vi "BASE_I_O_Screen.vi"(8 "error in (no error)":errorcluster) -> (0 "error out":errorcluster)   [LabVIEW 2017]
doc: "This vi is for manually turn ON and OFF also monitor Output of PLCS. So this is manual screen."
uses:
  <vilib>/Utility/file.llb/Read Delimited Spreadsheet (string).vi
  Global/PLC_to_Auto.vi
panel:
  out "CARD 8 OUTPUT":T1
  out "X27-SPARE 2":bool
  out "X26-SPARE 2":bool
  out "Y22 2":bool
  out "Y25":bool
  out "Y23":bool
  out "Y22":bool
  out "Y21":bool
  out "Y20-SPARE":bool
  out "X27-SPARE":bool
  out "X26-SPARE":bool
  out "X25-REJECTION FULL SENSOR":bool
  out "X24-REJECTION SENSOR":bool
  out "X23-DOOR 4":bool
  out "X22-DOOR 3":bool
  out "PART CLAMP END RS":bool
  out "UP DOWN CYL END RS":bool
  out "UP DOWN CYL  HM RS":bool
  out "PUSHER END RS":bool
  out "PUSHER HM RS":bool
  out "THREAD LOCKER CYL COMPLETE":bool
  out "SHUTTLE OPEN CHECK SENSOR-X300":bool
  out "SPARE":bool
  out "DOOR 2":bool
  out "DOOR 1":bool
  out "SAFETY SENSOR":bool
  out "GREEN LAMP":bool
  out "PRESSURE SWITCH":bool
  out "RESET PB":bool
  out "EMG STOP":bool
  out "CYCLE START TOUCH BUTTON 2":bool
  out "CYCLE START TOUCH BUTTON 1":bool
  out "BUZZER":bool
  out "RED LAMP":bool
  out "UP DN CYL REV SOL":bool
  out "UP DN CYL FWD SOL":bool
  out "PUSHER REV SOL":bool
  out "PUSHER FWD SOL":bool
  out "THREAD LOCKER OFF":bool
  out "THREAD LOCKER ON":bool
  out "PART CLAMP SOL":bool
  in  "Back":bool
  # "I/O Screen"
  # "OUTPUT"
  # "INPUT"
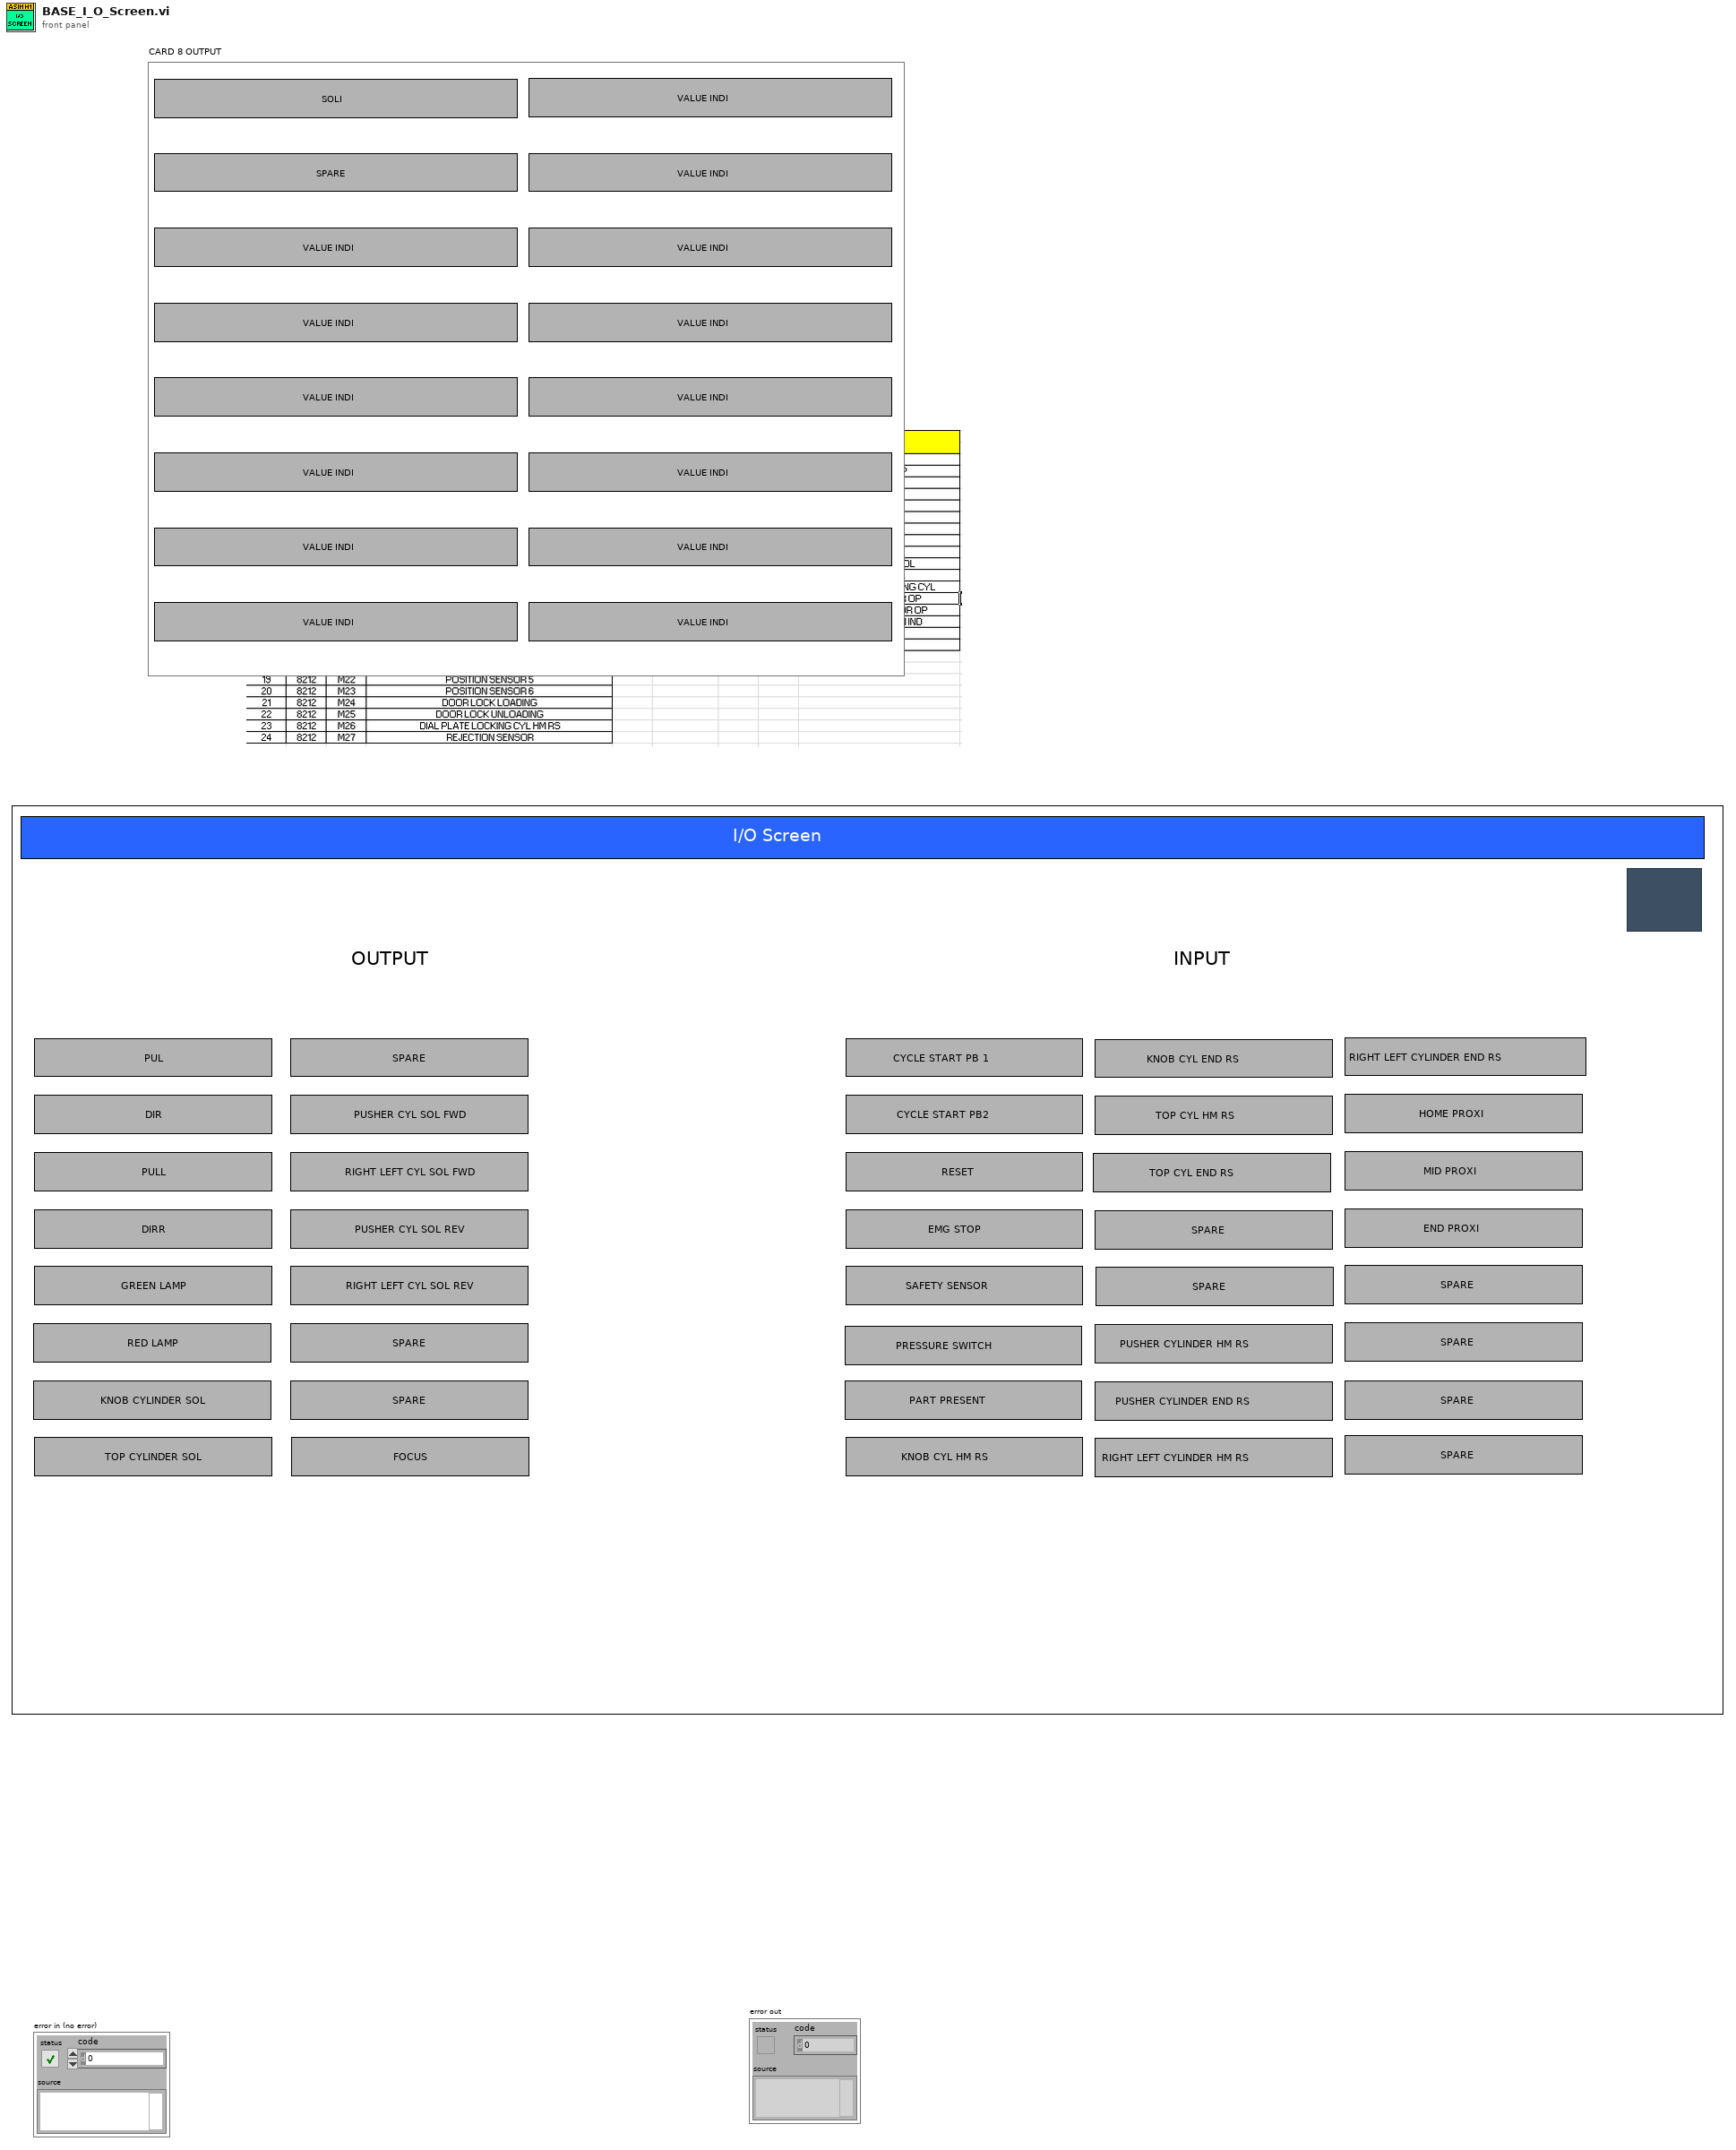
[diagram p1: front panel]
types:
  T1 = cluster{"8 CARD 1":bool, "8 CARD 2":bool, "8 CARD 3":bool, "8 CARD 4":bool, "8 CARD 5":bool, "8 CARD 6":bool, "8 CARD 7":bool, "8 CARD 8":bool, "8 CARD 9":bool, "8 CARD 10":bool, "8 CARD 11":bool, "8 CARD 12":bool, "8 CARD 13":bool, "8 CARD 14":bool, "8 CARD 15":bool, "8 CARD 16":bool}
  T2 = enum32{"invalid app kind", "Development System", "Run Time System", "Student Edition", "Embedded LabVIEW", "Evaluation", "Custom"}
  T3 = enum32{"Invalid", "Standard", "Closed", "Hidden", "Minimized", "Maximized"}
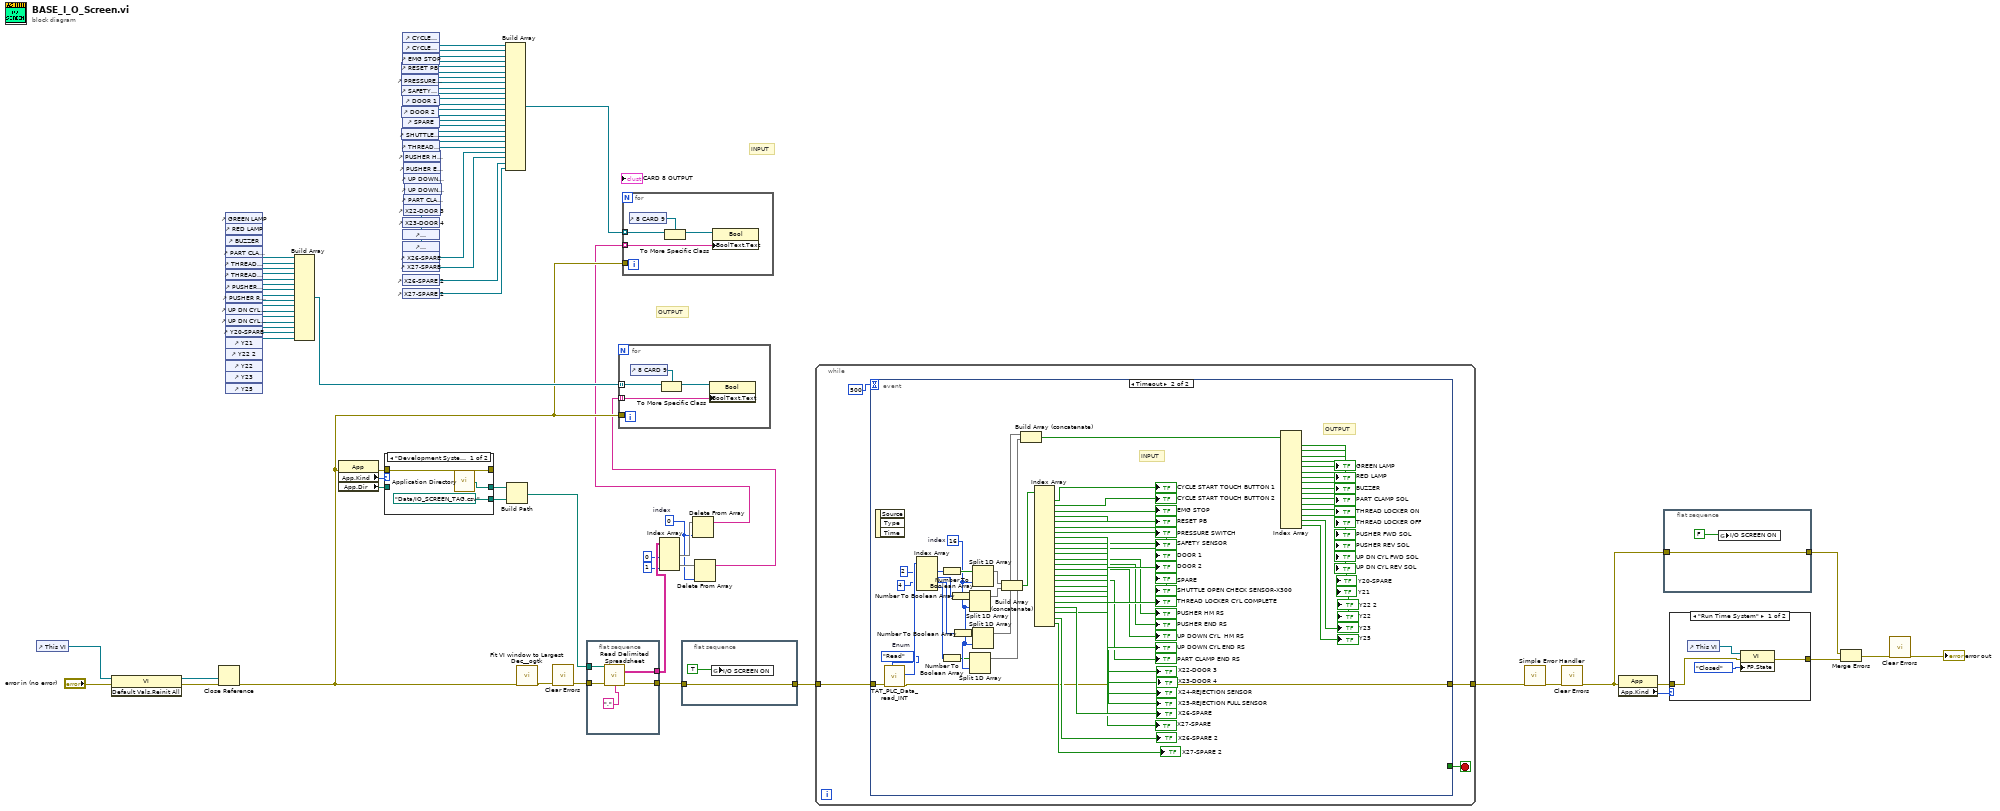
[diagram p0: block diagram]
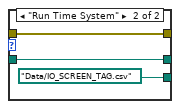
[diagram p2: hidden frame]
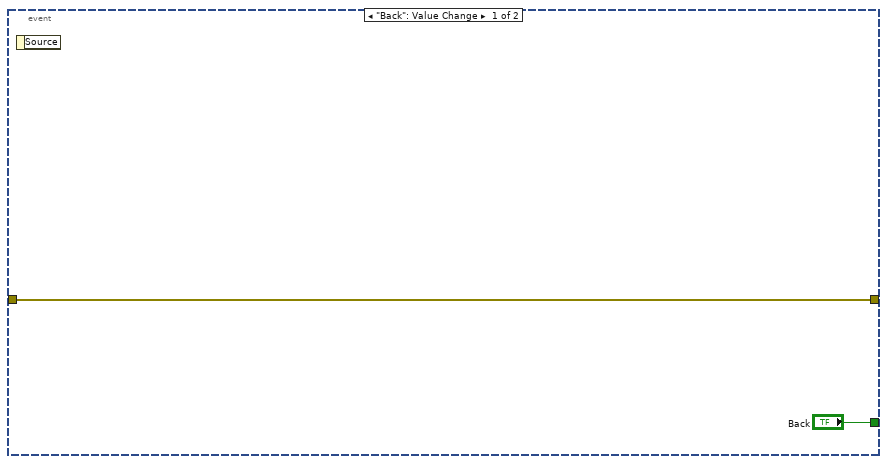
[diagram p4: hidden frame]
diagram:
  w55 = 0  # index
  # "OUTPUT"
  # "INPUT"
  n1 = control-ref of="This VI"() -> (w70:refnum<vi>)
  n2 = invoke class="VI" method="Default Vals.Reinit All"(reference=w70, error in="error in (no error)") -> (reference out=w68:refnum<vi>, error out=w67:errorcluster)  [unwired: 1 in, 1 out]
  n3 = Close Reference(reference=w68, error in (no error)=w67) -> (error out=w3:errorcluster)
  n4 = control-ref of="GREEN LAMP"() -> (w27:refnum<vi>)
  n5 = control-ref of="RED LAMP"() -> (w26:refnum<vi>)
  n6 = control-ref of="BUZZER"() -> (w25:refnum<vi>)
  n7 = control-ref of="PART CLAMP SOL"() -> (w24:refnum<vi>)
  n8 = control-ref of="THREAD LOCKER ON"() -> (w23:refnum<vi>)
  n9 = control-ref of="THREAD LOCKER OFF"() -> (w22:refnum<vi>)
  n10 = control-ref of="PUSHER FWD SOL"() -> (w21:refnum<vi>)
  n11 = control-ref of="PUSHER REV SOL"() -> (w20:refnum<vi>)
  n12 = control-ref of="UP DN CYL FWD SOL"() -> (w19:refnum<vi>)
  n13 = control-ref of="UP DN CYL REV SOL"() -> (w18:refnum<vi>)
  n14 = control-ref of="Y20-SPARE"() -> (w17:refnum<vi>)
  n15 = control-ref of="Y21"() -> (w16:refnum<vi>)
  n16 = control-ref of="Y22 2"() -> (w15:refnum<vi>)
  n17 = control-ref of="Y22"() -> (w14:refnum<vi>)
  n18 = control-ref of="Y23"() -> (w13:refnum<vi>)
  n19 = control-ref of="Y25"() -> (w12:refnum<vi>)
  n20 = Build Array(w27, w26, w25, w24, w23, w22, w21, w20, w19, w18, w17, w16, w15, w14, w13, w12) -> (w11:refnum<vi>[])
  n21 = property class="App"(error in=w3) -> (error out=w8:errorcluster, "App.Kind"=w6:T2, "App.Dir"=w7:path)  [unwired: 1 in, 1 out]
  n22 = case shown="\"Development System\", Default" w6 {
    tunnel: [w77 w80] -> _
    tunnel: w8 -> [w77 w80]
    tunnel: w7 -> [_ w79]
    tunnel: [w75 w79] -> w9
    tunnel: [path "Data/IO_SCREEN_TAG.csv" path "Data/IO_SCREEN_TAG.csv"] -> w10
    frame "Development System", Default {
      n23 = call <vilib>:"Application Directory.vi"() -> ("Application Directory"=w75:path)
    }
    frame "Run Time System" {
    }
  }
  n24 = control-ref of="SHUTTLE OPEN CHECK SENSOR-X300"() -> (w43:refnum<vi>)
  n25 = control-ref of="RESET PB"() -> (w49:refnum<vi>)
  n26 = control-ref of="PRESSURE SWITCH"() -> (w48:refnum<vi>)
  n27 = control-ref of="SAFETY SENSOR"() -> (w47:refnum<vi>)
  n28 = control-ref of="DOOR 2"() -> (w45:refnum<vi>)
  n29 = control-ref of="CYCLE START TOUCH BUTTON 1"() -> (w52:refnum<vi>)
  n30 = control-ref of="CYCLE START TOUCH BUTTON 2"() -> (w51:refnum<vi>)
  n31 = control-ref of="EMG STOP"() -> (w50:refnum<vi>)
  n32 = control-ref of="DOOR 1"() -> (w46:refnum<vi>)
  n33 = control-ref of="SPARE"() -> (w44:refnum<vi>)
  n34 = control-ref of="THREAD LOCKER CYL COMPLETE"() -> (w42:refnum<vi>)
  n35 = control-ref of="X23-DOOR 4"() -> (w35:refnum<vi>)
  n36 = control-ref of="X24-REJECTION SENSOR"() -> (w33:refnum<vi>)
  n37 = control-ref of="X25-REJECTION FULL SENSOR"() -> (w32:refnum<vi>)
  n38 = control-ref of="X26-SPARE"() -> (w31:refnum<vi>)
  n39 = control-ref of="X27-SPARE"() -> (w30:refnum<vi>)
  n40 = control-ref of="X26-SPARE 2"() -> (w29:refnum<vi>)
  n41 = control-ref of="X27-SPARE 2"() -> (w28:refnum<vi>)
  n42 = control-ref of="PUSHER HM RS"() -> (w41:refnum<vi>)
  n43 = control-ref of="PUSHER END RS"() -> (w40:refnum<vi>)
  n44 = control-ref of="X22-DOOR 3"() -> (w36:refnum<vi>)
  n45 = control-ref of="UP DOWN CYL  HM RS"() -> (w39:refnum<vi>)
  n46 = control-ref of="PART CLAMP END RS"() -> (w37:refnum<vi>)
  n47 = control-ref of="UP DOWN CYL END RS"() -> (w38:refnum<vi>)
  n48 = Build Array(w52, w51, w50, w49, w48, w47, w46, w45, w44, w43, w42, w41, w40, w39, w38, w37, w36, w35, w33, w32, w31, w30, w29, w28) -> (w34:refnum<vi>[])
  n49 = Build Path(base path=w9, name or relative path=w10) -> (appended path=w5:path)
  n50 = call <userlib>:"Fit VI window to Largest Dec__ogtk.vi"("error in (no error)"=w3) -> ("error out"=w53:errorcluster)  [unwired: 5 in, 1 out]
  n51 = call <vilib>:"Clear Errors.vi"("error in (no error)"=w53) -> ("error out"=w4:errorcluster)  [unwired: 5 in, 1 out]
  n52 = flat-sequence {
    tunnel: w4 -> [w84]
    tunnel: [w85] -> w54
    tunnel: w5 -> [w83]
    tunnel: [w81] -> w60
    frame #0 {
      n53 = call-poly <vilib>:"Read Delimited Spreadsheet.vi"("file path (dialog if empty)"=w83, "error in (no error)"=w84, "delimiter (\\t)"=",") -> ("all rows"=w81:string[][], "error out"=w85:errorcluster)  [unwired: 7 in, 4 out]
    }
  }
  n54 = Index Array(array=w60, index (col) #1=0, index (col) #2=1) -> (element #1=w57:string[], element #2=w56:string[])  [unwired: 2 in]
  n55 = flat-sequence {
    tunnel: w54 -> [w87]
    tunnel: [w87] -> w63
    frame #0 {
      n56 = global write "PLC_to_Auto.vi" "I/O SCREEN ON"(TRUE) -> ()
    }
  }
  n57 = Delete From Array(array=w57, index=w55) -> (array with subset deleted=w2:string[])  [unwired: 1 in, 1 out]
  n58 = for {
    tunnel: w2 -> [w89] mode=indexing
    tunnel: w34 -> [w88] mode=indexing
    tunnel: w3 -> [_]
    n59 = control-ref of="8 CARD 9"() -> (w90:refnum<vi>)
    n60 = To More Specific Class(target class=w90, reference=w88) -> (specific class reference=w91:refnum<vi>)  [unwired: 1 in, 1 out]
    n61 = property on="Property Node" class="Bool"(reference=w91, "BoolText.Text"=w89) -> ()  [unwired: 1 in, 2 out]
  }
  n62 = Delete From Array(array=w56, index=w55) -> (array with subset deleted=w1:string[])  [unwired: 1 in, 1 out]
  n63 = for {
    tunnel: w1 -> [w93] mode=indexing
    tunnel: w11 -> [w92] mode=indexing
    tunnel: w3 -> [_]
    n64 = control-ref of="8 CARD 9"() -> (w94:refnum<vi>)
    n65 = To More Specific Class(target class=w94, reference=w92) -> (specific class reference=w95:refnum<vi>)  [unwired: 1 in, 1 out]
    n66 = property on="Property Node" class="Bool"(reference=w95, "BoolText.Text"=w93) -> ()  [unwired: 1 in, 2 out]
  }
  n67 = while {
    tunnel: w63 -> [w99]
    tunnel: [w98] -> w73
    stop <- w97 stop-if-true
    n68 = event shown="[1] Timeout" {
      selector: _ -> [_ _]
      dyn-events: _ -> [_ _]
      timeout: 500 -> [_ _]
      tunnel: w99 -> [w100 w117]
      tunnel: [w100 w116] -> w98
      tunnel: ["Back" _] -> w97
      event "Back": Value Change {
        n69 = event-data() -> ()  [unwired: 1 in, 1 out]
      }
      event Timeout {
        w109 = 16  # index
        w118 = enum16{"Read", "Write"}."Read"  # Enum
        # "INPUT"
        # "OUTPUT"
        n70 = event-data() -> ()  [unwired: 1 in, 3 out]
        n71 = call "TAT_PLC_Data_read_INT.vi"("Enum"=w118, "error in (no error)"=w117) -> ("error out"=w116:errorcluster, "Array 2"=w122:u16[])  [unwired: 8 in]
        n72 = Index Array(array=w122, index #1=2, index #3=4) -> (element #1=w121:u16, element #2=w114:u16, element #3=w108:u16, element #4=w107:u16)  [unwired: 2 in]
        n73 = Number To Boolean Array(number=w121) -> (Boolean array=w120:bool[])
        n74 = Number To Boolean Array(number=w107) -> (Boolean array=w106:bool[])
        n75 = Number To Boolean Array(number=w114) -> (Boolean array=w115:bool[])
        n76 = Number To Boolean Array(number=w108) -> (Boolean array=w110:bool[])
        n77 = Split 1D Array(array=w115, index=w109) -> (first subarray=w111:bool[])  [unwired: 1 out]
        n78 = Split 1D Array(array=w106, index=w109) -> (first subarray=w104:bool[])  [unwired: 1 out]
        n79 = Split 1D Array(array=w120, index=w109) -> (first subarray=w113:bool[])  [unwired: 1 out]
        n80 = Split 1D Array(array=w110, index=w109) -> (first subarray=w105:bool[])  [unwired: 1 out]
        n81 = Build Array (concatenate)(w113, w111) -> (w112:bool[])
        n82 = Build Array (concatenate)(w105, w104) -> (w103:bool[])
        n83 = Index Array(array=w112) -> (element #1=→"CYCLE START TOUCH BUTTON 1":bool, element #2=→"CYCLE START TOUCH BUTTON 2":bool, element #3=→"EMG STOP":bool, element #4=→"RESET PB":bool, element #5=→"PRESSURE SWITCH":bool, element #6=→"SAFETY SENSOR":bool, element #7=→"DOOR 1":bool, element #8=→"DOOR 2":bool, element #9=→"SPARE":bool, element #10=→"SHUTTLE OPEN CHECK SENSOR-X300":bool, element #11=→"THREAD LOCKER CYL COMPLETE":bool, element #12=→"PUSHER HM RS":bool, element #13=→"PUSHER END RS":bool, element #14=→"UP DOWN CYL  HM RS":bool, element #15=→"UP DOWN CYL END RS":bool, element #16=→"PART CLAMP END RS":bool, element #17=→"X22-DOOR 3":bool, element #18=→"X23-DOOR 4":bool, element #19=→"X24-REJECTION SENSOR":bool, element #20=→"X25-REJECTION FULL SENSOR":bool, element #21=→"X26-SPARE":bool, element #22=→"X27-SPARE":bool, element #23=→"X26-SPARE 2":bool, element #24=→"X27-SPARE 2":bool)  [unwired: 24 in]
        n84 = Index Array(array=w103) -> (element #1=→"GREEN LAMP":bool, element #2=→"RED LAMP":bool, element #3=→"BUZZER":bool, element #4=→"PART CLAMP SOL":bool, element #5=→"THREAD LOCKER ON":bool, element #6=→"THREAD LOCKER OFF":bool, element #7=→"PUSHER FWD SOL":bool, element #8=→"PUSHER REV SOL":bool, element #9=→"UP DN CYL FWD SOL":bool, element #10=→"UP DN CYL REV SOL":bool, element #11=→"Y20-SPARE":bool, element #12=→"Y21":bool, element #13=→"Y22 2":bool, element #14=→"Y22":bool, element #15=→"Y23":bool, element #16=→"Y25":bool)  [unwired: 16 in]
      }
    }
  }
  n85 = call <vilib>:"Simple Error Handler.vi"("error in (no error)"=w73) -> ("error out"=w66:errorcluster)  [unwired: 4 in, 4 out]
  n86 = call <vilib>:"Clear Errors.vi"("error in (no error)"=w66) -> ("error out"=w62:errorcluster)  [unwired: 5 in, 1 out]
  n87 = property class="App"(error in=w62) -> (error out=w64:errorcluster, "App.Kind"=w65:T2)  [unwired: 1 in, 1 out]
  n88 = flat-sequence {
    tunnel: w62 -> [w164]
    tunnel: [w164] -> w61
    frame #0 {
      n89 = global write "PLC_to_Auto.vi" "I/O SCREEN ON"(FALSE) -> ()
    }
  }
  n90 = case shown="\"Run Time System\"" w65 {
    tunnel: w64 -> [w166 w169]
    tunnel: [w165 w169] -> w71
    frame "Run Time System" {
      n91 = control-ref of="This VI"() -> (w168:refnum<vi>)
      n92 = property class="VI"(reference=w168, error in=w166, "FP.State"=T3."Closed" ("Front Panel Window:State")) -> (error out=w165:errorcluster)  [unwired: 1 out]
    }
    frame "Development System", Default {
    }
  }
  n93 = Merge Errors(w61, w71) -> (w72:errorcluster)
  n94 = call <vilib>:"Clear Errors.vi"("error in (no error)"=w72) -> ("error out"=→"error out":errorcluster)  [unwired: 5 in, 1 out]
